vi "ACT_NTS.vi"(1 "number IN":u8 format="%.0x") -> (0 "string OUT":string)   [LabVIEW 2011]
doc: "Author: Roberto ORSELLO\nDate: January 2007\nDescription: subroutine that converts a U8 decimal number\nto a string number that can be used to write one single Byte to\nany VISA device"
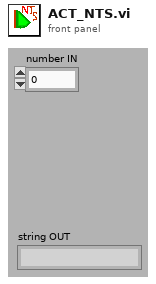
[diagram p1: front panel]
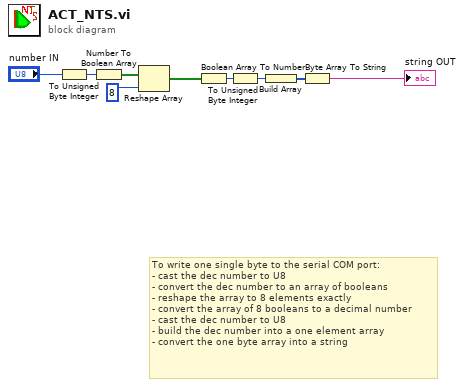
[diagram p0: block diagram]
diagram:
  # "To write one single byte to the serial COM port:\n- cast the dec number to U8\n- convert the dec number to an array of booleans\n- reshape the array to 8 elements exactly\n- convert the array of 8 booleans to a decimal number\n- cast the dec number to U8\n- build the dec number into a one element array\n- convert the one byte array into a string"
  n1 = To Unsigned Byte Integer(number="number IN") -> (unsigned 8bit integer=w2:u8)
  n2 = Number To Boolean Array(number=w2) -> (Boolean array=w7:bool[])
  n3 = Reshape Array(w7, 8 ("dimension size")) -> (w1:bool[])
  n4 = Boolean Array To Number(Boolean array=w1) -> (number=w5:u32)
  n5 = To Unsigned Byte Integer(number=w5) -> (unsigned 8bit integer=w4:u8)
  n6 = Build Array(w4) -> (w3:u8[])
  n7 = Byte Array To String(unsigned byte array=w3) -> (string=→"string OUT":string)
